vi "Test Filters.vi"() -> ()   [LabVIEW 2019]
uses:
  src/subVIs/Zero Phase Lowpass Filter (multiple).vi
  src/subVIs/Savitsky Golay Filter (multiple).vi
  src/subVIs/Moving Average (multiple).vi
  src/subVIs/Zero Phase Lowpass Filter (single).vi
  src/subVIs/Savitsky Golay Filter (single).vi
  src/subVIs/Moving Average (single).vi
  src/Private/Get X Array dx.vi
  src/Private/X Units.vi
  <vilib>/Analysis/3filter.llb/Savitzky-Golay Filter.vi
  <vilib>/Analysis/3filter.llb/Savitzky-Golay Filter (DBL).vi
  src/Private/X Array Range to Index.vi
  <vilib>/Analysis/3filter.llb/FIR Windowed Coefficients.vi
  <vilib>/Analysis/3filter.llb/Zero Phase Filter.vi
  <vilib>/Analysis/3filter.llb/Zero Phase Filter (DBL).vi
  <vilib>/Utility/error.llb/Error Cluster From Error Code.vi
  <vilib>/Analysis/3filter.llb/Smoothing Filter Coefficients.vi
  <vilib>/Analysis/3filter.llb/IIR Filter.vi
  <vilib>/Analysis/3filter.llb/IIR Filter (DBL).vi
  src/xy_utilities.lvlib
panel:
  out "Intensity Graph 2":dbl[][](graph)
  out "Intensity Graph":dbl[][](graph)
  in  "parameter":dbl
  in  "Dataset":T1(ring)=enum."superlattice waveguide"
  in  "index":i32
  out "XY Data Filtered 2":cluster{"X-array":dbl[], "Y-array":dbl[]}[](graph)
  in  "Filter":enum16{"Lowpass", "SG", "Moving"}(ring)
  out "execution time (s)":dbl
  out "XY Data Filtered":cluster{"X-array":dbl[], "Y-array":dbl[]}[](graph)
  out "XY Data":cluster{"X-array":dbl[], "Y-array":dbl[]}[](graph)
  # "0: 21\"\n5: 0.09\""
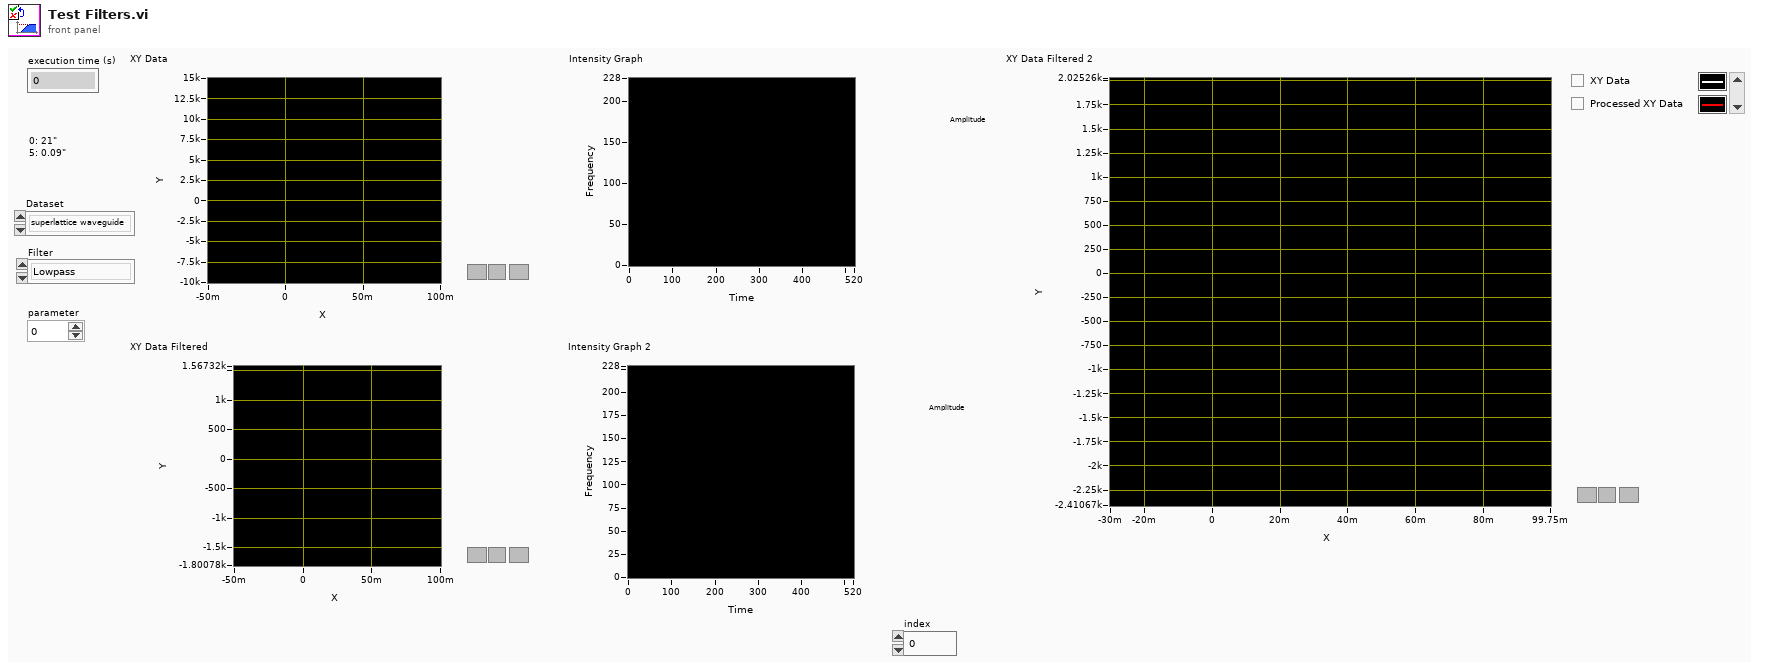
[diagram p1: front panel]
types:
  T1 = enum16{"thermal waveguide", "superlattice waveguide", "decay in atmosphere"}
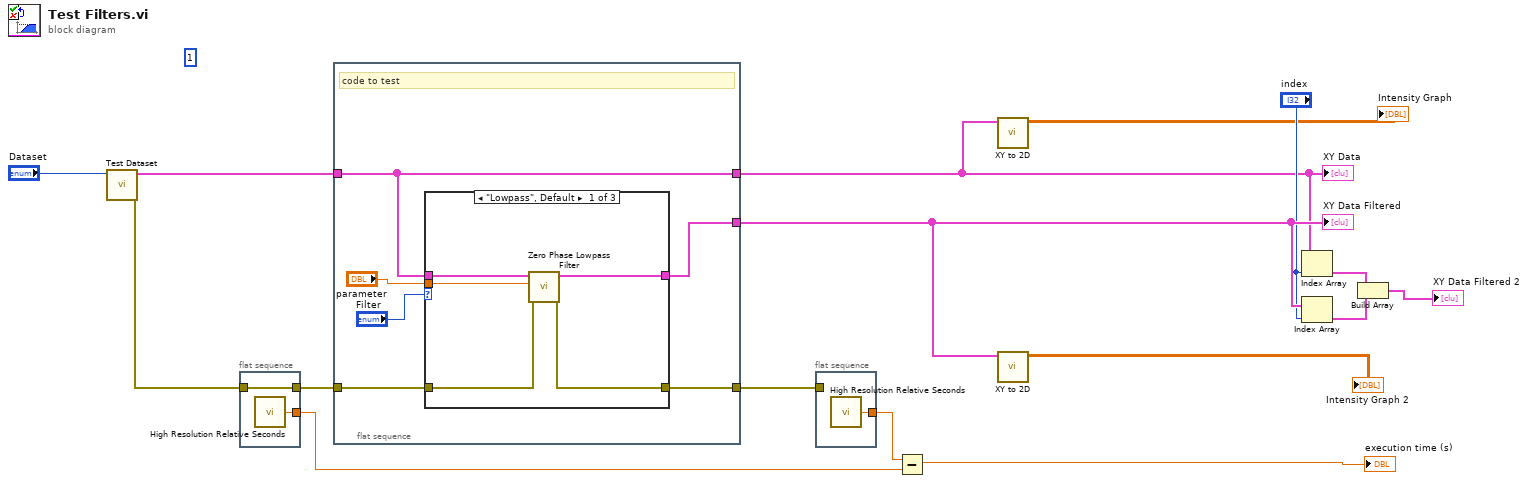
[diagram p0: block diagram]
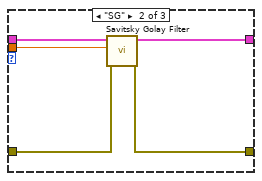
[diagram p2: hidden frame]
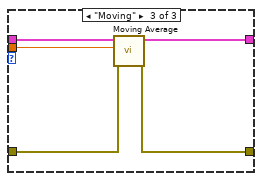
[diagram p3: hidden frame]
diagram:
  (unwired) 1
  n1 = call "Test Dataset.vi"("Enum"="Dataset") -> ("error out"=w16:errorcluster, "XY-data out"=w15:cluster{"X-array":dbl[], "Y-array":dbl[]}[])  [unwired: 8 in, 1 out]
  n2 = flat-sequence {
    tunnel: [w18] -> w5
    tunnel: w16 -> [w18]
    tunnel: [w17] -> w6
    frame #0 {
      n3 = call <vilib>:"High Resolution Relative Seconds.vi"() -> ("relative seconds"=w17:dbl)
    }
  }
  n4 = flat-sequence {
    tunnel: w15 -> [w24]
    tunnel: [w23] -> w13
    tunnel: w5 -> [w22]
    tunnel: [w21] -> w4
    tunnel: [w24] -> w3
    frame #0 {
      # "code to test"
      n5 = case shown="\"Lowpass\", Default" "Filter" {
        tunnel: w24 -> [w29 w34 w39]
        tunnel: [w28 w33 w38] -> w23
        tunnel: w22 -> [w27 w32 w37]
        tunnel: [w26 w31 w36] -> w21
        tunnel: "parameter" -> [w25 w30 w35]
        frame "Lowpass", Default {
          n6 = call-poly "Zero Phase Lowpass Filter.vi"("error in (no error)"=w27, "cutoff period (data)"=w25, "XY-data"=w29) -> ("error out"=w26:errorcluster, "XY-data out"=w28:cluster{"X-array":dbl[], "Y-array":dbl[]}[])  [unwired: 7 in]
        }
        frame "SG" {
          n7 = call-poly "Savitsky Golay Filter.vi"("error in (no error)"=w32, "side points"=w30, "XY-data"=w34) -> ("error out"=w31:errorcluster, "XY-data out"=w33:cluster{"X-array":dbl[], "Y-array":dbl[]}[])  [unwired: 7 in]
        }
        frame "Moving" {
          n8 = call-poly "Moving Average.vi"("error in (no error)"=w37, "Window"=w35, "XY-data"=w39) -> ("error out"=w36:errorcluster, "XY-data out"=w38:cluster{"X-array":dbl[], "Y-array":dbl[]}[])  [unwired: 7 in]
        }
      }
    }
  }
  n9 = flat-sequence {
    tunnel: [w40] -> w7
    tunnel: w4 -> [_]
    frame #0 {
      n10 = call <vilib>:"High Resolution Relative Seconds.vi"() -> ("relative seconds"=w40:dbl)
    }
  }
  n11 = Subtract(x=w7, y=w6) -> (x-y=→"execution time (s)":dbl)
  n12 = call "XY to 2D.vi"("XY-data"=w3) -> ("2D Y Array"=→"Intensity Graph":dbl[][])  [unwired: 7 in, 3 out]
  n13 = call "XY to 2D.vi"("XY-data"=w13) -> ("2D Y Array"=→"Intensity Graph 2":dbl[][])  [unwired: 7 in, 3 out]
  n14 = Index Array(array=w3, index="index") -> (element=w11:cluster{"X-array":dbl[], "Y-array":dbl[]})
  n15 = Index Array(array=w13, index="index") -> (element=w12:cluster{"X-array":dbl[], "Y-array":dbl[]})
  n16 = Build Array(w11, w12) -> (→"XY Data Filtered 2":cluster{"X-array":dbl[], "Y-array":dbl[]}[])
  "XY Data" <- w3
  "XY Data Filtered" <- w13
